vi "PVCAM_CloseCamera.vi"(8 "error in (no error)":errorcluster, 11 "hCam":i16) -> (0 "error out":errorcluster, 2 "return type 2":i16)   [LabVIEW 2021]
uses:
  pvcam64.dll
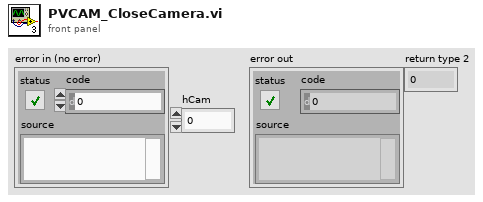
[diagram p1: front panel]
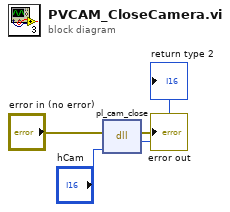
[diagram p0: block diagram]
diagram:
  n1 = dll-call lib="pvcam64.dll" fn="pl_cam_close"(error in="error in (no error)", "hCam"="hCam") -> (error out=→"error out":errorcluster, "return type"=→"return type 2":i16)  [unwired: 3 in, 1 out]
